vi "Merge alignment.vi"(8 "Image info":T3(array[cluster])=[{"File name"=path "\\\\jg-i\\c-drive/LabView development/Glimpse/Test Data/Merge test/gelles00089.tif", "TIFF stack?"=TRUE, "Frame # if stack?"=1}, {"File name"=path "\\\\jg-i\\c-drive/LabView development/Glimpse/Test Data/Merge test/gelles00089.tif", "TIFF stack?"=TRUE, "Frame # if stack?"=1}]) -> (1 "Display info out":T2(array[cluster]), 3 "Image info Out":T3(array[cluster])=[{"File name"=path "\\\\jg-i\\c-drive/LabView development/Glimpse/Test Data/Merge test/gelles00096full.tif", "TIFF stack?"=TRUE, "Frame # if stack?"=1}, {"File name"=path "\\\\jg-i\\c-drive/LabView development/Glimpse/Test Data/Merge test/gelles00097full.tif", "TIFF stack?"=TRUE, "Frame # if stack?"=1}])   [LabVIEW 2011]
doc: "Loads the images being used to select control points and run the Matlab control point selection tool to allow the user to pick the points."
uses:
  <vilib>/vision/Image Controls.llb/IMAQ Image.ctl
  GLIMPSE Globals.vi
  <vilib>/vision/NI_Vision_Development_Module.lvlib
panel:
  in  "1. Continue after setting file names":bool
  in  "2. Continue after setting B/W":bool
  in  "Stop":bool
  # "Be sure to use ³2 control point pairs for linear conformal; ³3 for affine; \nand ³4 for projective."
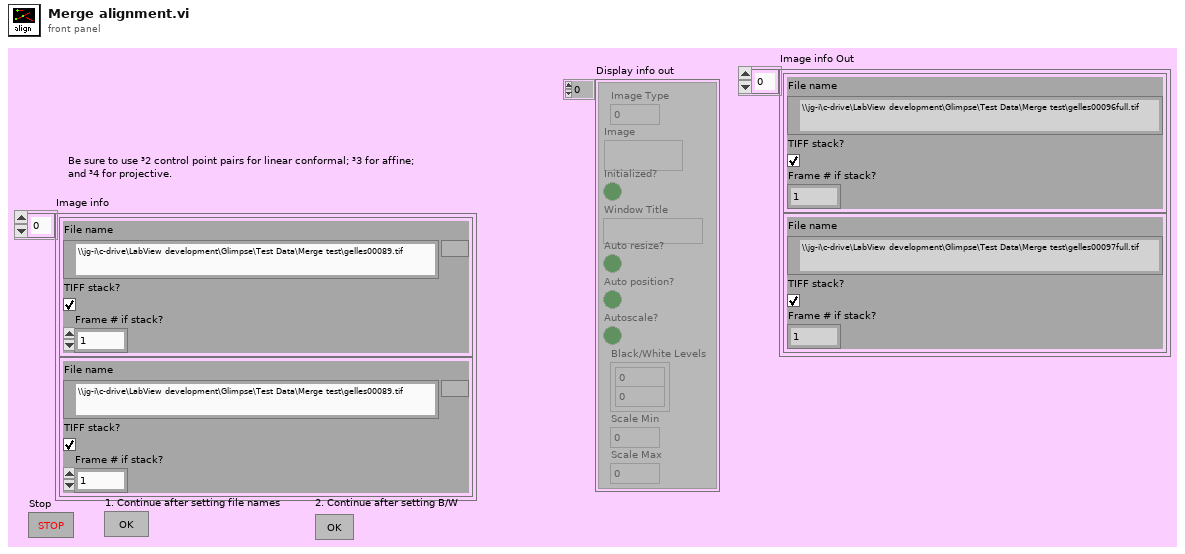
[diagram p1: front panel]
types:
  T1 = typedef "IMAQ Image.ctl" = refnum<image>
  T2 = cluster{"Image Type":u32, "Image":T1, "Initialized?":bool, "Window Title":string, "Auto resize?":bool, "Auto position?":bool, "Autoscale?":bool, "Black/White Levels":cluster{ext, ext}, "Scale Min":ext, "Scale Max":ext}[]
  T3 = cluster{"File name":path, "TIFF stack?":bool, "Frame # if stack?":u32}[]
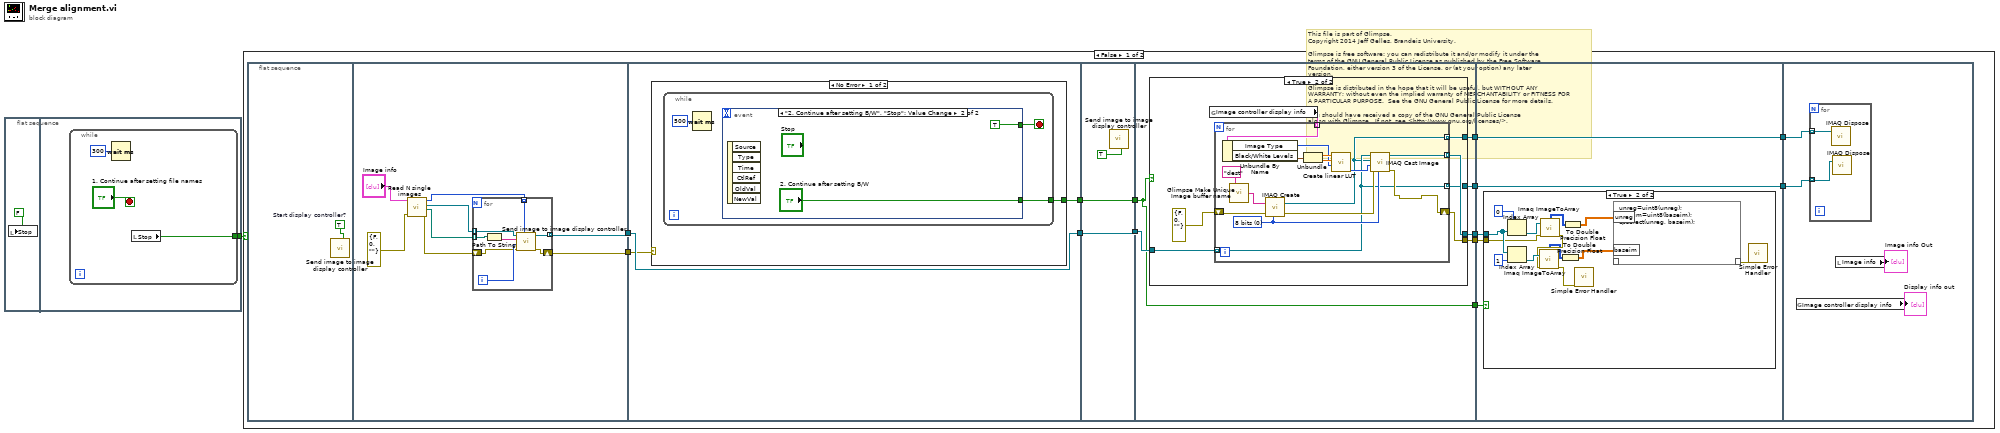
[diagram p0: block diagram]
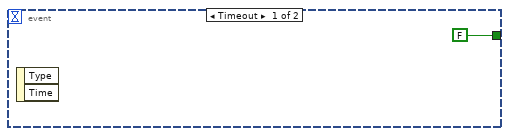
[diagram p2: hidden frame]
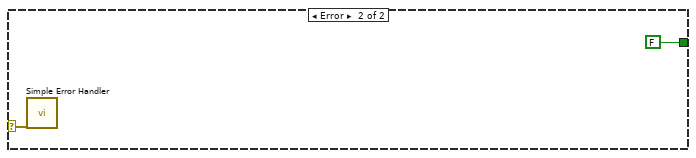
[diagram p3: hidden frame]
diagram:
  # "This file is part of Glimpse. \nCopyright 2014 Jeff Gelles, Brandeis University.    \n\nGlimpse is free software: you can redistribute it and/or modify it under the \nterms of the GNU General Public License as published by the Free Software \nFoundation, either version 3 of the License, or (at your option) any later \nversion.\n\nGlimpse is distributed in the hope that it will be useful, but WITHOUT ANY \nWARRANTY; without even the implied warranty of MERCHANTABILITY or FITNESS FOR \nA PARTICULAR PURPOSE.  See the GNU General Public License for more details.\n\nYou should have received a copy of the GNU General Public License\nalong with Glimpse.  If not, see <http://www.gnu.org/licenses/>."
  n1 = flat-sequence {
    tunnel: [w3] -> w1
    frame #0 {
      n2 = local write "Stop"(FALSE ("stop")) -> ()
    }
    frame #1 {
      n3 = while {
        tunnel: [w4] -> w3
        stop <- "1. Continue after setting file names" stop-if-true
        n4 = Wait (ms)(milliseconds to wait=u32 300) -> ()  [unwired: 1 out]
        n5 = local read "Stop"() -> (w4:bool)
      }
    }
  }
  n6 = case shown="False" w1 {
    frame False {
      n7 = flat-sequence {
        tunnel: [w26] -> w19
        tunnel: [w22] -> w18
        tunnel: w19 -> [w39]
        tunnel: [w39] -> w17
        tunnel: [w38] -> w16
        tunnel: w18 -> [w37]
        tunnel: w17 -> [w51]
        tunnel: [w51] -> w15
        tunnel: w16 -> [w49]
        tunnel: [w49] -> w14
        tunnel: w15 -> [w57]
        tunnel: [w56] -> w13
        tunnel: [w55] -> w12
        tunnel: [w54] -> w11
        tunnel: [w53] -> w10
        tunnel: w14 -> [w52]
        tunnel: [w52] -> w9
        tunnel: w13 -> [w85]
        tunnel: w12 -> [w84]
        tunnel: [w84] -> w8
        tunnel: w11 -> [w83]
        tunnel: [w83] -> w7
        tunnel: w10 -> [w82]
        tunnel: w9 -> [w81]
        tunnel: w8 -> [w102]
        tunnel: w7 -> [w101]
        frame #0 {
          w20 = TRUE  # Start display controller?
          n8 = call "Send image to image display controller.vi"("Start display controller?"=w20) -> ()  [unwired: 6 in, 4 out]
        }
        frame #1 {
          n9 = call "Read N single images.vi"("error in"=errorcluster {"status"=FALSE, "code"=0, "source"=""} ("error out"), "Image info"="Image info") -> ("error out"=w25:errorcluster, "File paths out"=w24:path[], "Images out"=w23:T1[], "Image types out"=w21:u32[])  [unwired: 4 out]
          n10 = for {
            tunnel: [w35] -> w26 mode=indexing
            shift-right: [w34] -> w22
            shift-left: w25 -> [w30]
            tunnel: w24 -> [w32] mode=indexing
            tunnel: w23 -> [w31] mode=indexing
            tunnel: w21 -> [w29] mode=indexing
            i -> [w33]
            n11 = Path To String(path=w32) -> (string=w36:string)
            n12 = call "Send image to image display controller.vi"("Image"=w31, "Window Title"=w36, "Window Number"=w33, "error in"=w30, "Image Type"=w29) -> ("Image Out"=w35:T1, "error out"=w34:errorcluster)  [unwired: 2 in, 2 out]
          }
        }
        frame #2 {
          n13 = case shown="No Error" w37 {
            selector: w37 -> [_ w47]
            tunnel: [w40 FALSE ("Continue after setting B/W")] -> w38
            frame No Error {
              n14 = while {
                tunnel: [w41] -> w40
                stop <- w42 stop-if-true
                n15 = Wait (ms)(milliseconds to wait=u32 500) -> ()  [unwired: 1 out]
                n16 = event shown="[1] \"2. Continue after setting B/W\", \"Stop\": Value Change" {
                  selector: _ -> [_ _]
                  dyn-events: _ -> [_ _]
                  timeout: _ -> [_ _]
                  tunnel: [FALSE TRUE] -> w42
                  tunnel: [_ "2. Continue after setting B/W"] -> w41
                  event Timeout {
                    n17 = event-data() -> ()  [unwired: 3 out]
                  }
                  event "2. Continue after setting B/W", "Stop": Value Change {
                    n18 = event-data() -> ()  [unwired: 7 out]
                  }
                }
              }
            }
            frame Error {
              n19 = call <vilib>:"Simple Error Handler.vi"("error in (no error)"=w47) -> ()  [unwired: 1 in, 8 out]
            }
          }
        }
        frame #3 {
          n20 = call "Send image to image display controller.vi"("Quit display controller?"=TRUE) -> ()  [unwired: 6 in, 4 out]
        }
        frame #4 {
          n21 = case shown="True" w52 {
            tunnel: w57 -> [w58 w63]
            tunnel: [_ w62] -> w56
            tunnel: [w58 w61] -> w55
            tunnel: [_ w60] -> w54
            tunnel: [_ w59] -> w53
            frame False {
            }
            frame True {
              n22 = global read "GLIMPSE Globals.vi" "Image controller display info"() -> (w65:T2)
              n23 = for {
                tunnel: w63 -> [w67] mode=indexing
                tunnel: w65 -> [w80] mode=indexing
                shift-right: [w68] -> w59
                shift-left: errorcluster {"status"=FALSE, "code"=0, "source"=""} ("error out") -> [w71]
                tunnel: [w70] -> w62 mode=indexing
                tunnel: [w67] -> w61 mode=indexing
                tunnel: [w66] -> w60 mode=indexing
                w69 = u32 0 items=["8 bits", "16 bits", "Float", "Complex", "RGB", "HSL"] ("Image Type")
                n24 = Unbundle By Name(w80) -> ("Image Type"=w76:u32, "Black/White Levels"=w79:cluster{ext, ext})
                n25 = call "Glimpse Make Unique Image buffer name.vi"("Buffer  base name"="dest") -> ("Image Name"=w74:string)  [unwired: 1 out]
                n26 = call "IMAQ Create"("Image Name"=w74, "Image Type"=w69, "error in (no error)"=w71) -> ("New Image"=w66:T1, "error out"=w72:errorcluster)  [unwired: 1 in, 1 out]
                n27 = Unbundle(w79) -> (w78:ext, w77:ext)
                n28 = call "Create linear LUT.vi"("Input Image Type"=w76, "White Value"=w77, "Black Value"=w78) -> ("LUT (U8) Out"=w75:u8[])  [unwired: 6 out]
                n29 = call "IMAQ Cast Image"("Image Type"=w69, "error in (no error)"=w72, "Lookup Table"=w75, "Image Dst"=w66, "Image Src"=w67) -> ("error out"=w68:errorcluster, "Image Dst Out"=w70:T1)  [unwired: 1 in, 4 out]
              }
            }
          }
        }
        frame #5 {
          n30 = case shown="True" w81 {
            tunnel: w85 -> [_ w90]
            tunnel: w82 -> [_ w86]
            frame False {
            }
            frame True {
              n31 = Index Array(array=w90, index=0) -> (element=w95:T1)
              n32 = Index Array(array=w90, index=1) -> (element=w94:T1)
              n33 = call "Imaq ImageToArray"("error in (no error)"=w86, "Image"=w95) -> ("error out"=w93:errorcluster, "Image Pixels (U8)"=w88:u8[][])  [unwired: 1 in, 4 out]
              n34 = call "Imaq ImageToArray"("error in (no error)"=w93, "Image"=w94) -> ("error out"=w89:errorcluster, "Image Pixels (U8)"=w87:u8[][])  [unwired: 1 in, 4 out]
              n35 = To Double Precision Float(number=w87) -> (double precision float=w97:dbl[][])
              n36 = To Double Precision Float(number=w88) -> (double precision float=w96:dbl[][])
              n37 = call <vilib>:"Simple Error Handler.vi"("error in (no error)"=w89) -> ()  [unwired: 1 in, 8 out]
              n38 = script code="unreg=uint8(unreg);\nbaseim=uint8(baseim);\ncpselect(unreg, baseim);"("baseim"=w97, "unreg"=w96) -> ("??"=w98:errorcluster)  [unwired: 1 out]
              n39 = call <vilib>:"Simple Error Handler.vi"("error in (no error)"=w98) -> ()  [unwired: 1 in, 8 out]
            }
          }
        }
        frame #6 {
          n40 = global read "GLIMPSE Globals.vi" "Image controller display info"() -> (→"Display info out":T2)
          n41 = for {
            tunnel: w102 -> [w104] mode=indexing
            tunnel: w101 -> [w103] mode=indexing
            n42 = call "IMAQ Dispose"("Image"=w103) -> ()  [unwired: 2 in, 4 out]
            n43 = call "IMAQ Dispose"("Image"=w104) -> ()  [unwired: 2 in, 4 out]
          }
          n44 = local read "Image info"() -> (→"Image info Out":T3)
        }
      }
    }
    frame True {
    }
  }
